vi "Bootloader - Check Filename And Update Device.vi"(0 "VISA resource name":refnum<visa-resource-name>, 1 ".X settings":T1={"reg. address"=82, "address content (en)"=82, "address content (dis)"=82, "fw .hex file path"=path "Fir", "updater path"=path "Fir"}, 2 "Device has .X":bool, 7 "device name":string, 11 "current versions":u8[](array[numeric])) -> (4 "VISA resource name":refnum<visa-resource-name>, 15 "error out":errorcluster)   [LabVIEW 2010]
uses:
  <vilib>/Utility/sysdir.llb/System Directory Type.ctl
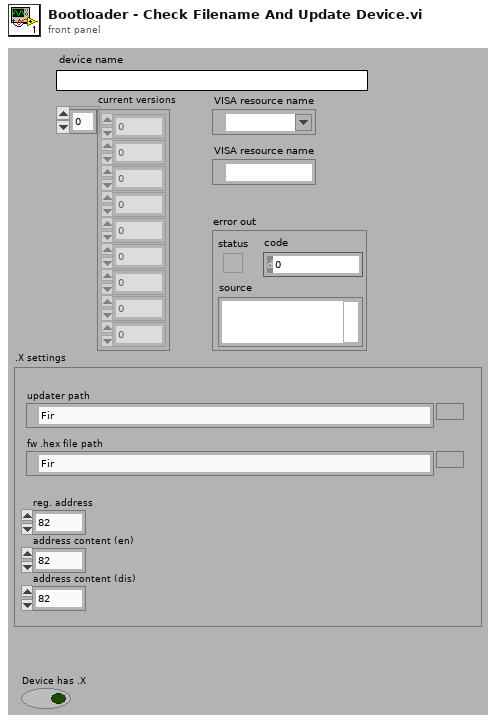
[diagram p1: front panel]
types:
  T1 = cluster{"reg. address":u8, "address content (en)":u8, "address content (dis)":u8, "fw .hex file path":path, "updater path":path}
  T2 = typedef "System Directory Type.ctl" = i32
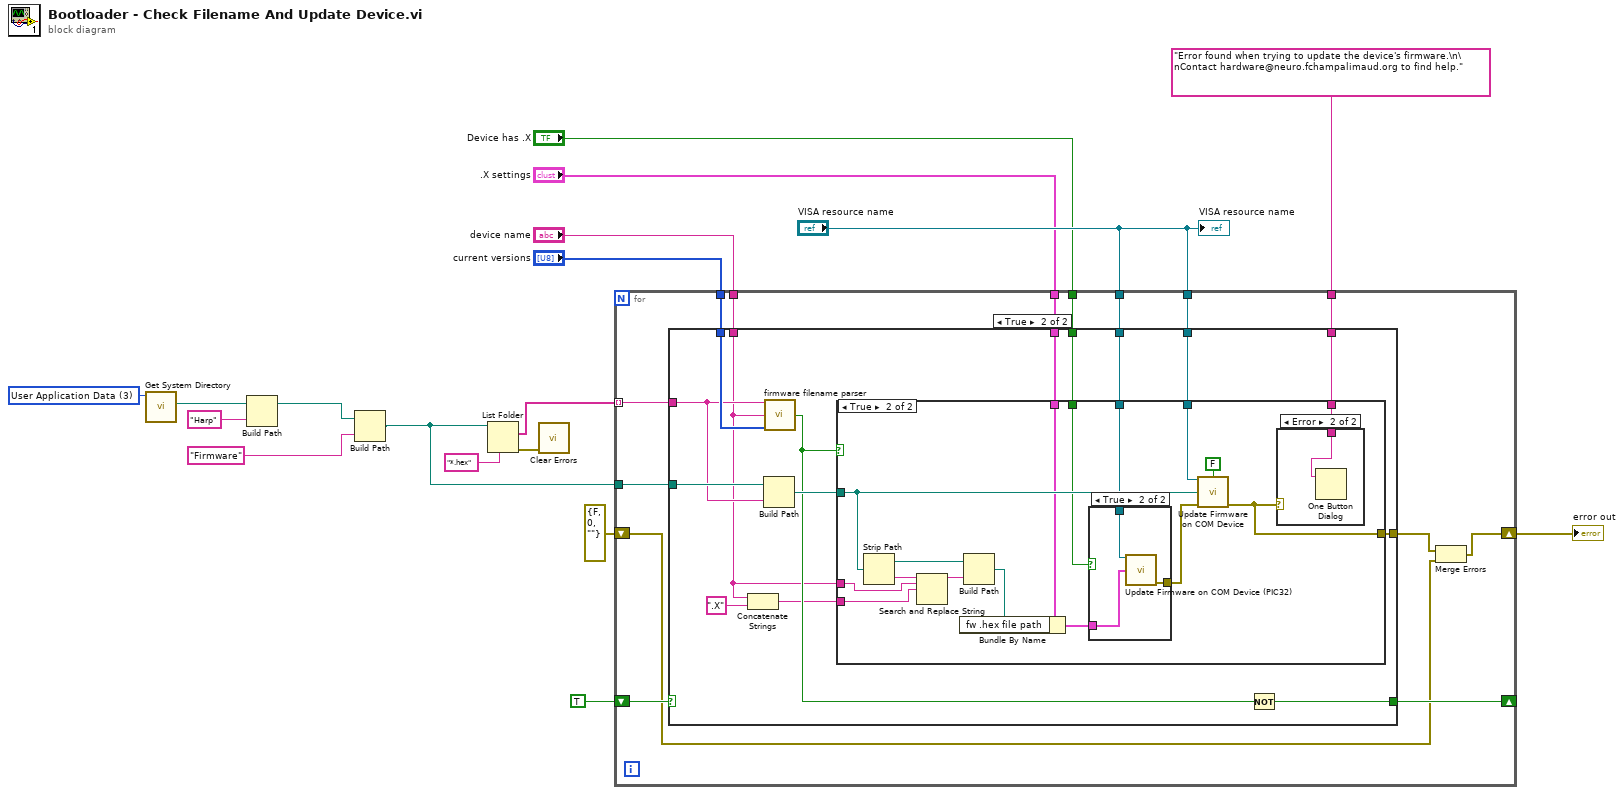
[diagram p0: block diagram]
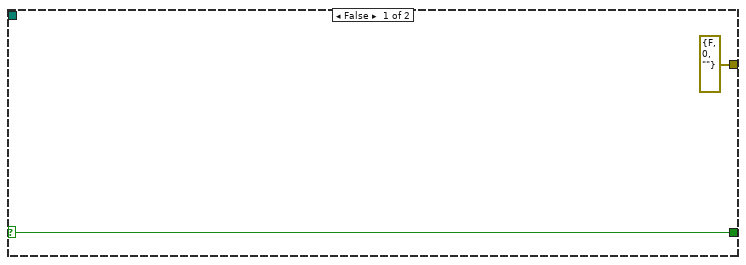
[diagram p2: hidden frame]
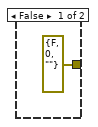
[diagram p3: hidden frame]
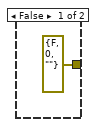
[diagram p4: hidden frame]
diagram:
  w11 = T2 3 items=["User Home"=0, "User Desktop"=1, "User Documents"=2, "User Application Data"=3, "User Preferences"=4, "User Temporary"=5, "Public Documents"=6, "Public Application Data"=7, "Public Preferences"=8, "Public Cache"=13, "System Core Libraries"=9, "System Installed Libraries"=10, "Application Files"=11, "Boot Volume Root"=12] ("system directory type")
  n1 = call <vilib>:"Get System Directory.vi"("system directory type"=w11) -> ("system directory"=w10:path)  [unwired: 10 in]
  n2 = Build Path(base path=w10, name or relative path="Harp") -> (appended path=w9:path)
  n3 = Build Path(base path=w9, name or relative path="Firmware") -> (appended path=w7:path)
  n4 = List Folder(path=w7, pattern="*.hex") -> (filenames=w16:string[], error out=w17:errorcluster)  [unwired: 2 in, 2 out]
  n5 = call <vilib>:"Clear Errors.vi"("error in (no error)"=w17) -> ()  [unwired: 6 in, 1 out]
  n6 = for {
    tunnel: w16 -> [w29] mode=indexing
    tunnel: "device name" -> [w32]
    tunnel: "current versions" -> [w31]
    tunnel: w7 -> [w30]
    shift-right: [w27] -> _
    shift-left: TRUE -> [w28]
    tunnel: "VISA resource name" -> [w26]
    shift-right: [w24] -> w6
    shift-left: errorcluster {"status"=FALSE, "code"=0, "source"=""} ("error IO") -> [w23]
    tunnel: "Error found when trying to update the device's firmware.\n\nContact hardware@neuro.fchampalimaud.org to find help." ("message") -> [w22]
    tunnel: ".X settings" -> [w21]
    tunnel: "VISA resource name" -> [w20]
    tunnel: "Device has .X" -> [w19]
    n7 = case shown="True" w28 {
      selector: w28 -> [w34 _]
      tunnel: w32 -> [_ w39]
      tunnel: w31 -> [_ w49]
      tunnel: w30 -> [_ w48]
      tunnel: w29 -> [_ w47]
      tunnel: [w34 w44] -> w27
      tunnel: w26 -> [_ w43]
      tunnel: [errorcluster {"status"=FALSE, "code"=0, "source"=""} ("error out") w42] -> w25
      tunnel: w22 -> [_ w41]
      tunnel: w21 -> [_ w40]
      tunnel: w20 -> [_ w36]
      tunnel: w19 -> [_ w35]
      frame False {
      }
      frame True {
        n8 = Concatenate Strings(w39, ".X" ("string")) -> (w37:string)
        n9 = Build Path(base path=w48, name or relative path=w47) -> (appended path=w46:path)
        n10 = call "firmware filename parser.vi"("filename"=w47, "firmware name"=w39, "current versions"=w49) -> ("update firmware"=w45:bool)  [unwired: 12 in]
        n11 = case shown="True" w45 {
          tunnel: w46 -> [_ w62]
          tunnel: w43 -> [_ w65]
          tunnel: [errorcluster {"status"=FALSE, "code"=0, "source"=""} ("error out") w64] -> w42
          tunnel: w41 -> [_ w63]
          tunnel: w40 -> [_ w56]
          tunnel: w39 -> [_ w60]
          tunnel: w37 -> [_ w59]
          tunnel: w36 -> [_ w53]
          tunnel: w35 -> [_ w52]
          frame False {
          }
          frame True {
            n12 = Strip Path(path=w62) -> (stripped path=w58:path, name=w61:string)
            n13 = Search and Replace String(input string=w61, search string=w60, replace string=w59) -> (result string=w57:string)  [unwired: 5 in, 3 out]
            n14 = Build Path(base path=w58, name or relative path=w57) -> (appended path=w55:path)
            n15 = Bundle By Name(cluster=w56, "fw .hex file path"=w55) -> (w51:T1)
            n16 = case shown="True" w52 {
              tunnel: [errorcluster {"status"=FALSE, "code"=0, "source"=""} ("error out") w70] -> w54
              tunnel: w51 -> [_ w69]
              tunnel: w53 -> [_ w68]
              frame False {
              }
              frame True {
                n17 = call "Update Firmware on COM Device (PIC32).vi"("VISA resource name"=w68, ".X settings"=w69) -> ("error out"=w70:errorcluster)  [unwired: 13 in]
              }
            }
            n18 = call "Update Firmware on COM Device.vi"("VISA resource name"=w65, "Skip Bootloader call"=FALSE, ".hex path"=w62, "error in (no error)"=w54) -> ("error out"=w64:errorcluster)  [unwired: 11 in]
            n19 = case shown="Error" w64 {
              tunnel: w63 -> [_ w71]
              frame No Error {
              }
              frame Error {
                n20 = One Button Dialog(message=w71) -> ()  [unwired: 1 in, 1 out]
              }
            }
          }
        }
        n21 = Not(x=w45) -> (.not. x?=w44:bool)
      }
    }
    n22 = Merge Errors(w25, w23) -> (w24:errorcluster)
  }
  "error out" <- w6
  "VISA resource name" <- "VISA resource name"
